vi "ingest_video.vi"(7 "Timestamp Manifest":refnum<class "timestampManifest.lvclass">, 8 "error in":errorcluster, 9 "Target":refnum<class "target.lvclass">, 10 "Source":refnum<class "source.lvclass">, 11 "Nominal Client in":refnum<class "Nominal Client.lvclass">) -> (0 "error out":errorcluster, 1 "videoFileRid":string, 2 "videoRid":string, 3 "Nominal Client out":refnum<class "Nominal Client.lvclass">)   [LabVIEW 2020, in "Nominal Client.lvclass"]
doc: "Triggers an ingest job, allowing either creating a new dataset or uploading to an existing one. This endpoint is meant to supersede all other ingestion endpoints as their functionality gets migrated to this one."
uses:
  Nominal Client.lvclass
  datasources/target/target.lvclass
  datasources/source/source.lvclass
  nominal types/timestampManifest/timestampManifest/timestampManifest.lvclass
  Nominal Client.lvclass/Nominal Client.ctl
  datasources/target/target.lvclass/target.ctl
  7ecb1b1c-631a-4c89-b8b8-2ed88685cfb3.vi
  datasources/target/workspace.set.vi
  <vilib>/JDP Science/JSONtext/support/Format JSON Object.vi
  <vilib>/JDP Science/JSONtext/JSON text to Variant.vi
  <vilib>/JDP Science/JSONtext/LVClass Serializer/JSONtext LVClass Serializer.lvclass
  <vilib>/JDP Science/JSONtext/JSONtext.lvlib
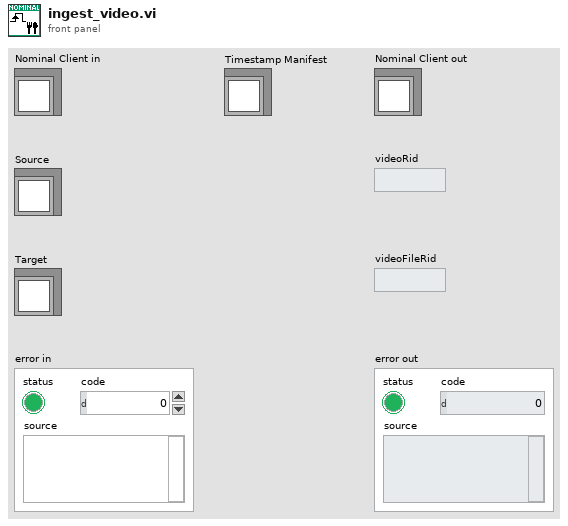
[diagram p1: front panel]
types:
  T1 = cluster{"details":cluster{"type":string, "video":cluster{"videoFileRid":string, "videoRid":string}}}
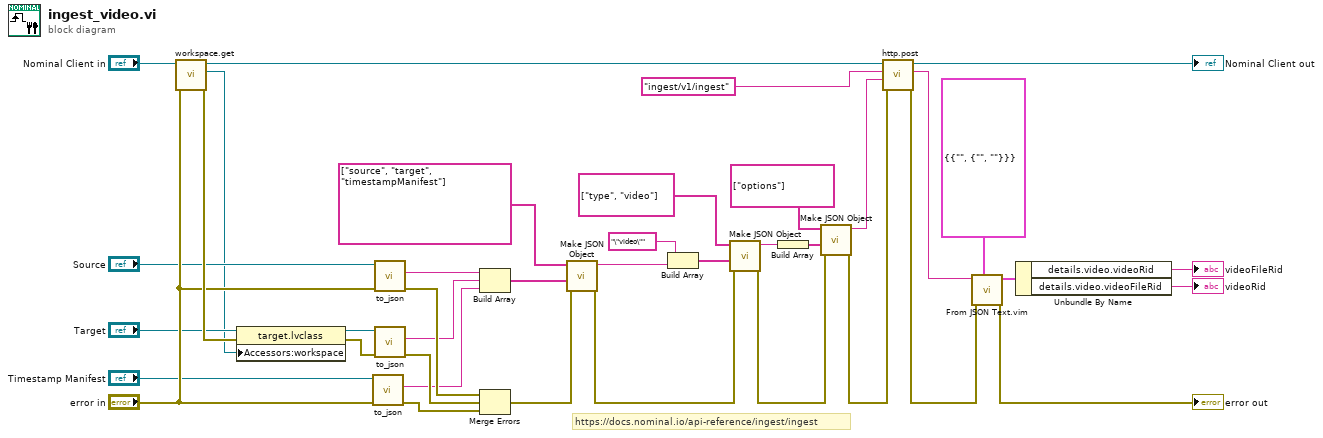
[diagram p0: block diagram]
diagram:
  # "https://docs.nominal.io/api-reference/ingest/ingest"
  n1 = call "workspace.get.vi"("error in"="error in", "Nominal Client in"="Nominal Client in") -> ("error out"=w27:errorcluster, "workspace"=w10:refnum<class "workspace.lvclass">, "Nominal Client out"=w32:refnum<class "Nominal Client.lvclass">)  [unwired: 7 in]
  n2 = property class="target.lvclass"(reference="Target", error in=w27, "Accessors:workspace"=w10) -> (reference out=w34:refnum<class "target.lvclass">, error out=w35:errorcluster)
  n3 = call-dynamic "to_json.vi"("error in"="error in", "timestampManifest in"="Timestamp Manifest") -> ("error out"=w26:errorcluster, "json"=w29:string)  [unwired: 6 in, 2 out]
  n4 = call-dynamic "to_json.vi"("error in"="error in", "source in"="Source") -> ("error out"=w37:errorcluster, "json"=w31:string)  [unwired: 6 in, 2 out]
  n5 = call-dynamic "to_json.vi"("error in"=w35, "target in"=w34) -> ("error out"=w36:errorcluster, "json"=w30:string)  [unwired: 6 in, 2 out]
  n6 = Build Array(w31, w30, w29) -> (w22:string[])
  n7 = Merge Errors(w37, w36, w26) -> (w28:errorcluster)
  n8 = call <vilib>:"Make JSON Object.vi"("error in (no error)"=w28, "JSON Items"=w22, "Item Names"=string[] ["source", "target", "timestampManifest"]) -> ("error out"=w17:errorcluster, "<JSON>"=w18:string)  [unwired: 7 in]
  n9 = Build Array("\"video\"" ("JSON"), w18) -> (w20:string[])
  n10 = call <vilib>:"Make JSON Object.vi"("error in (no error)"=w17, "JSON Items"=w20, "Item Names"=string[] ["type", "video"] ("JSON")) -> ("error out"=w5:errorcluster, "<JSON>"=w7:string)  [unwired: 7 in]
  n11 = Build Array(w7) -> (w8:string[])
  n12 = call <vilib>:"Make JSON Object.vi"("error in (no error)"=w5, "JSON Items"=w8, "Item Names"=string[] ["options"] ("JSON")) -> ("error out"=w4:errorcluster, "<JSON>"=w6:string)  [unwired: 7 in]
  n13 = call "http.post.vi"("error in"=w4, "Request body"=w6, "Path"="ingest/v1/ingest", "Nominal Client in"=w32) -> ("error out"=w13:errorcluster, "Response"=w14:string, "Nominal Client out"=→"Nominal Client out":refnum<class "Nominal Client.lvclass">)  [unwired: 4 in, 1 out]
  n14 = call "From JSON Text.vim"("Data Type and Default Value"=T1 {"details"={"type"="", "video"={"videoFileRid"="", "videoRid"=""}}}, "error in (no error)"=w13, "JSON"=w14) -> ("error out"=→"error out":errorcluster, "Data out"=w11:T1)  [unwired: 7 in]
  n15 = Unbundle By Name(w11) -> ("details.video.videoRid"=→"videoFileRid":string, "details.video.videoFileRid"=→"videoRid":string)
